vi "String splitter step.vi"(0 "Input string":string, 1 "regular expression 1":string=";", 2 "regular expression 2":string="=|>|<") -> (19 "Condition value 3":dbl, 20 "Condition name 1":string, 21 "Condition comparator 1":string, 22 "Condition value 1":dbl, 23 "Condition name 2":string, 24 "Condition comparator 2":string, 25 "Condition value 2":dbl, 26 "Condition name 3":string, 27 "Condition comparator 3":string)   [LabVIEW 2014]
uses:
  <vilib>/regexp/Match Regular Expression.xnode
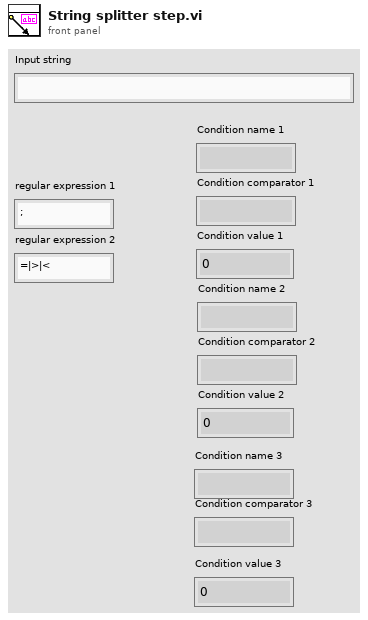
[diagram p1: front panel]
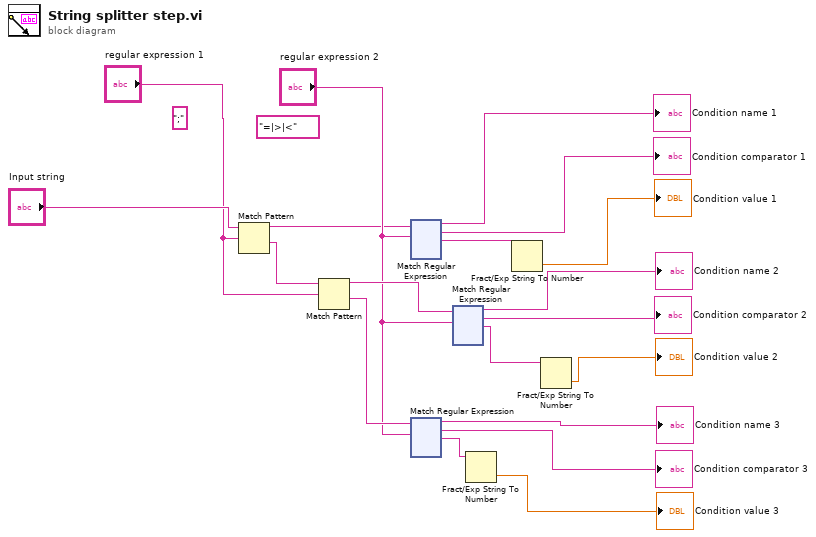
[diagram p0: block diagram]
diagram:
  (unwired) "=|>|<" ("regular expression")
  (unwired) ";" ("regular expression")
  n1 = Match Pattern(string="Input string", regular expression="regular expression 1") -> (before substring=w1:string, after substring=w19:string)  [unwired: 1 in, 2 out]
  n2 = Match Pattern(string=w19, regular expression="regular expression 1") -> (before substring=w18:string, after substring=w17:string)  [unwired: 1 in, 2 out]
  n3 = xnode "Match Regular Expression"("input string"=w1, "regular expression"="regular expression 2") -> ("before match"=→"Condition name 1":string, "whole match"=→"Condition comparator 1":string, "after match"=w14:string)  [unwired: 4 in, 2 out]
  n4 = xnode "Match Regular Expression"("input string"=w17, "regular expression"="regular expression 2") -> ("before match"=→"Condition name 3":string, "whole match"=→"Condition comparator 3":string, "after match"=w12:string)  [unwired: 4 in, 2 out]
  n5 = xnode "Match Regular Expression"("input string"=w18, "regular expression"="regular expression 2") -> ("before match"=→"Condition name 2":string, "whole match"=→"Condition comparator 2":string, "after match"=w13:string)  [unwired: 4 in, 2 out]
  n6 = Fract/Exp String To Number(string=w12) -> (number=→"Condition value 3":dbl)  [unwired: 3 in, 1 out]
  n7 = Fract/Exp String To Number(string=w14) -> (number=→"Condition value 1":dbl)  [unwired: 3 in, 1 out]
  n8 = Fract/Exp String To Number(string=w13) -> (number=→"Condition value 2":dbl)  [unwired: 3 in, 1 out]
